vi "Open.vi"(8 "error in (no error)":errorcluster, 11 "TXT_Writer in":refnum<class "TXT_Writer.lvclass">) -> (0 "error out":errorcluster, 3 "TXT_Writer out":refnum<class "TXT_Writer.lvclass">)   [LabVIEW 2024, in "Data.lvlib" / "TXT_Writer.lvclass"]
uses:
  TXT_Writer.lvclass
  C:/Users/aheme/Documents/Dev/DEV_INFO/DEV_INFO/StockM/MyLabVIEW_Framework/Data/DataWriter/DataWriter.lvclass
  TXT_Writer.lvclass/TXT_Writer.ctl
  Data/DataWriter/DataWriter.lvclass/DataWriter.ctl
  Data/DataWriter/DataWriter.lvclass
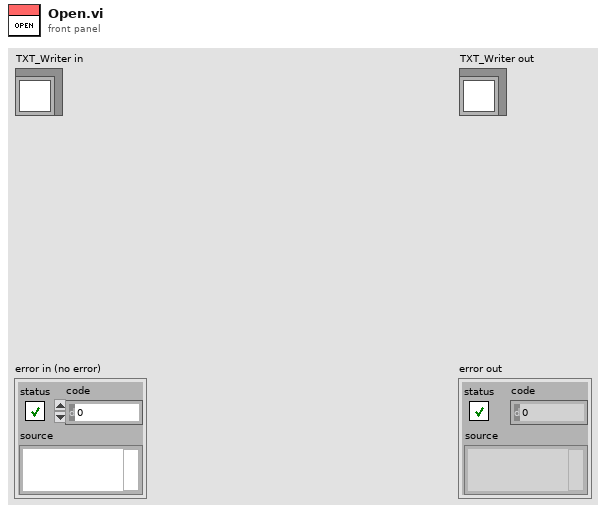
[diagram p1: front panel]
types:
  T1 = enum16{"open", "replace", "create", "open or create", "replace or create", "replace or create with confirmation"}
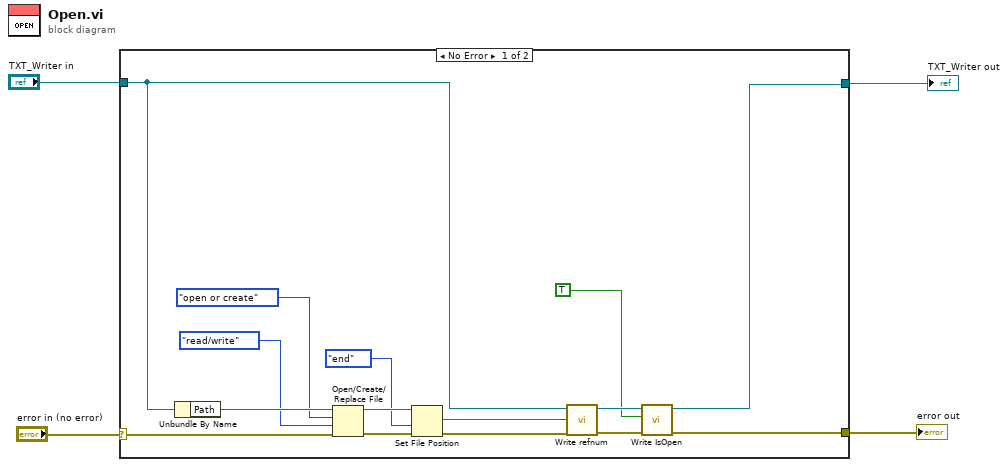
[diagram p0: block diagram]
diagram:
  n1 = case shown="No Error" "error in (no error)" {
    selector: "error in (no error)" -> [w18 w21]
    tunnel: [w16 w21] -> w4
    tunnel: [w12 w20] -> w3
    tunnel: "TXT_Writer in" -> [w17 w20]
    frame No Error {
      n2 = Unbundle By Name(w17) -> ("Path"=w19:path)
      n3 = Open/Create/Replace File(file path (use dialog)=w19, error in=w18, operation (0:open)=T1."open or create", access (0:read/write)=enum16{"read/write", "read-only", "write-only"}."read/write") -> (refnum out=w9:refnum<file>, error out=w8:errorcluster)  [unwired: 2 in, 1 out]
      n4 = Set File Position(refnum=w9, from (0:start)=enum16{"start", "end", "current"}."end", error in=w8) -> (refnum out=w5:refnum<file>, error out=w7:errorcluster)  [unwired: 1 in]
      n5 = call "Write refnum.vi"("error in (no error)"=w7, "refnum"=w5, "DataWriter in"=w17) -> ("error out"=w15:errorcluster, "DataWriter out"=w14:refnum<class "TXT_Writer.lvclass">)  [unwired: 7 in]
      n6 = call "Write IsOpen.vi"("error in (no error)"=w15, "IsOpen"=TRUE, "DataWriter in"=w14) -> ("error out"=w16:errorcluster, "DataWriter out"=w12:refnum<class "TXT_Writer.lvclass">)  [unwired: 7 in]
    }
    frame Error {
    }
  }
  "error out" <- w4
  "TXT_Writer out" <- w3
